vi "Read Measurement (Burst Interval).vi"(0 "VISA resource name":refnum<visa-resource-name>, 5 "Source (0: Channel 1)":i32(ring) items=["Channel 1", "Channel 2", "Channel 3", "Channel 4", "Function 1", "Function 2", "Function 3", "Function 4", "Memory 1", "Memory 2", "Memory 3", "Memory 4"], 7 "Idle Time (0)":dbl, 9 "Maximum Time (10000ms)":u32=10000, 11 "error in (no error)":errorcluster) -> (4 "VISA resource name out":refnum<visa-resource-name>, 10 "Burst Interval Time":dbl, 15 "error out":errorcluster)   [LabVIEW 2020, in "Agilent 90000 Series.lvlib"]
doc: "Returns the amount of time between the end of a burst and beginning of the next burst."
uses:
  Agilent 90000 Series.lvlib
  Low Level/Fetch Measurement (Burst Interval).vi
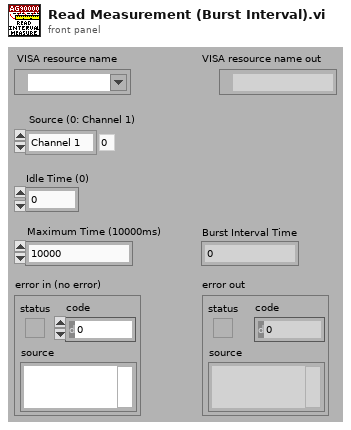
[diagram p1: front panel]
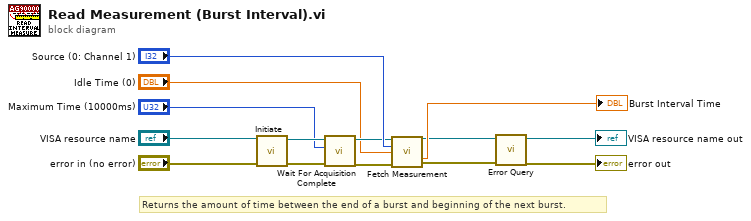
[diagram p0: block diagram]
diagram:
  # "Returns the amount of time between the end of a burst and beginning of the next burst."
  n1 = call "Initiate.vi"("error in (no error)"="error in (no error)", "VISA resource name"="VISA resource name") -> ("error out"=w12:errorcluster, "VISA resource name out"=w11:refnum<visa-resource-name>)  [unwired: 8 out]
  n2 = call "Wait For Acquisition Complete.vi"("error in (no error)"=w12, "Maximum Time (10000ms)"="Maximum Time (10000ms)", "VISA resource name"=w11) -> ("error out"=w4:errorcluster, "VISA resource name out"=w5:refnum<visa-resource-name>)  [unwired: 7 out]
  n3 = call-poly "Fetch Measurement.vi"("VISA resource name"=w5, "Source (0: Channel 1)"="Source (0: Channel 1)", "Idle Time (0)"="Idle Time (0)", "error in (no error)"=w4) -> ("VISA resource name out"=w3:refnum<visa-resource-name>, "Burst Interval Time"=→"Burst Interval Time":dbl, "error out"=w2:errorcluster)  [unwired: 1 in, 8 out]
  n4 = call "Error Query.vi"("error in (no error)"=w2, "VISA resource name"=w3) -> ("error out"=→"error out":errorcluster, "VISA resource name out"=→"VISA resource name out":refnum<visa-resource-name>)  [unwired: 1 in, 7 out]
